vi "Create Colour.vi"(6 "B":u8, 8 "error in (no error)":errorcluster, 9 "G":u8, 10 "R":u8, 11 "Surface Pointer":u32 format="%.0x") -> (0 "error out":errorcluster, 3 "Colour":u32 format="%.0x")   [LabVIEW 2015, in "LibSDL2.lvlib"]
doc: "Uses the surface to determine the correct pixel format."
uses:
  LibSDL2.lvlib
  SDL2 Utility/SDL2 Utility.lvlib
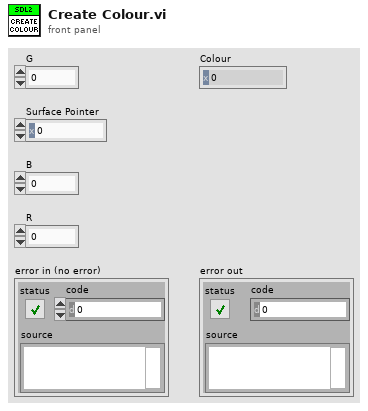
[diagram p1: front panel]
types:
  T1 = typedef "LibSDL2.lvlib/Surface.ctl" = cluster{"Flags":u32, "Pixel Format Pointer":u32, "Width":i32, "Height":i32, "Pitch":i32, "Pixels Pointer":u32, "User Data Pointer":u32, "Locked":i32, "Lock Data Pointer":u32, "Clip Rectangle":T2, "Blitmap Pointer":u32, "Ref Count":i32}
  T2 = typedef "LibSDL2.lvlib/Rectangle.ctl" = cluster{"x":i32, "y":i32, "Width":i32, "Height":i32}
  T3 = typedef "LibSDL2.lvlib/Pixel Formal.ctl" = cluster{"Format":u32, "Palette Pointer":u32, "BitsPerPixel":u8, "BytesPerPixel":u8, "Padding 1":u8, "Padding 2":u8, "Rmask":u32, "Gmask":u32, "Bmask":u32, "Amask":u32, "Rloss":u8, "Gloss":u8, "Bloss":u8, "Aloss":u8, "Rshift":u8, "Gshift":u8, "Bshift":u8, "Ashift":u8, "Ref Count":i32, "Next Pointer":u32}
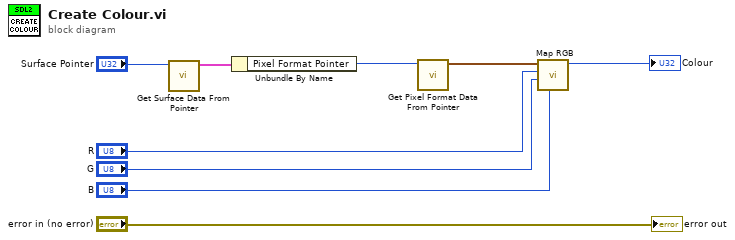
[diagram p0: block diagram]
diagram:
  n1 = call "Get Surface Data From Pointer.vi"("Surface Pointer"="Surface Pointer") -> ("Surface Data"=w3:T1)  [unwired: 9 in, 1 out]
  n2 = Unbundle By Name(w3) -> ("Pixel Format Pointer"=w2:u32)
  n3 = call "Get Pixel Format Data From Pointer.vi"("Pixel Format Pointer"=w2) -> ("Data"=w6:T3)  [unwired: 9 in, 1 out]
  n4 = call "Map RGB.vi"("B"="B", "G"="G", "R"="R", "Pixel Format"=w6) -> ("Colour"=→"Colour":u32)  [unwired: 6 in, 1 out]
  "error out" <- "error in (no error)"
